vi "Shaped Pulse Train Test.vi"() -> ()   [LabVIEW 2015]
uses:
  Waveform VIs/Shaped Pulse Train VIs/SPT-Properties.ctl
  Waveform VIs/Shaped Pulse Train VIs/SPT-Shape.ctl
panel:
  out "Waveform Graph":dbl[](graph)
  in  "Fs":dbl
  in  "SPT.Properties":T1
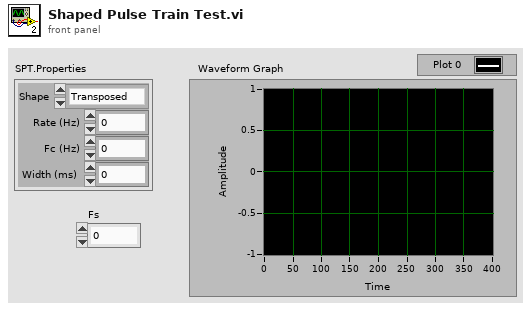
[diagram p1: front panel]
types:
  T1 = typedef "SPT-Properties.ctl" = cluster{"Shape":T2, "Rate (Hz)":dbl, "Fc (Hz)":dbl, "Width (ms)":dbl}
  T2 = typedef "SPT-Shape.ctl" = enum16{"Transposed", "Alpha", "Gabor"}
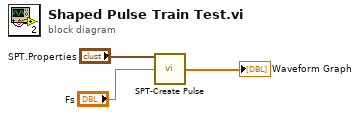
[diagram p0: block diagram]
diagram:
  n1 = call "SPT-Create Pulse.vi"("SPT.Properties"="SPT.Properties", "Fs (Hz)"="Fs") -> ("Pulse"=→"Waveform Graph":dbl[])  [unwired: 12 in, 1 out]
